vi "Set - wForm from Raw Data.vi"(0 "reference in":refnum<class "GSwFormDSP.lvclass">, 5 "error in (no error)":errorcluster, 6 "X Unit":string, 7 "Y Data (Row matrix)":dbl[][](array[numeric]), 8 "Data Origin":string, 9 "dTs":dbl[](array[numeric]), 10 "Signal Set":T1(ring), 11 "Signals Name":string[](array[string]), 13 "Signals Unit":string[](array[string])) -> (14 "reference in":refnum<class "GSwFormDSP.lvclass">, 19 "error out":errorcluster)   [LabVIEW 2020, in "GSwFormDSP.lvclass"]
uses:
  GSwFormDSP.lvclass
  functions/Attribute List.ctl
  Generic Utilities_class/Generic Utilities.lvclass
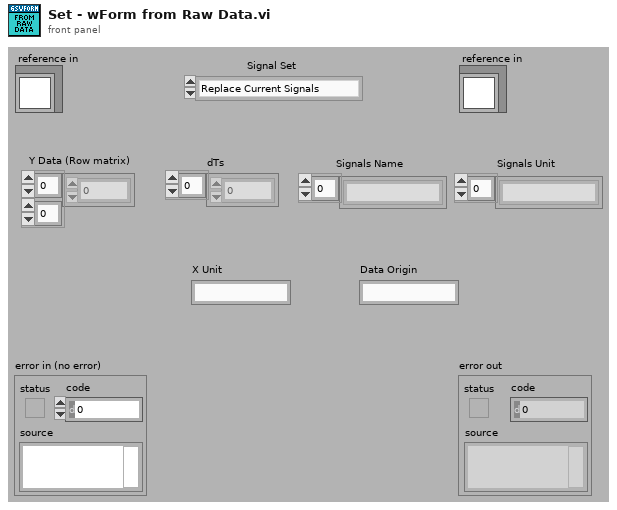
[diagram p1: front panel]
types:
  T1 = enum16{"Replace Current Signals", "Append to Current Signals"}
  T2 = typedef "GSwFormDSP.lvclass/Attribute List.ctl" = string
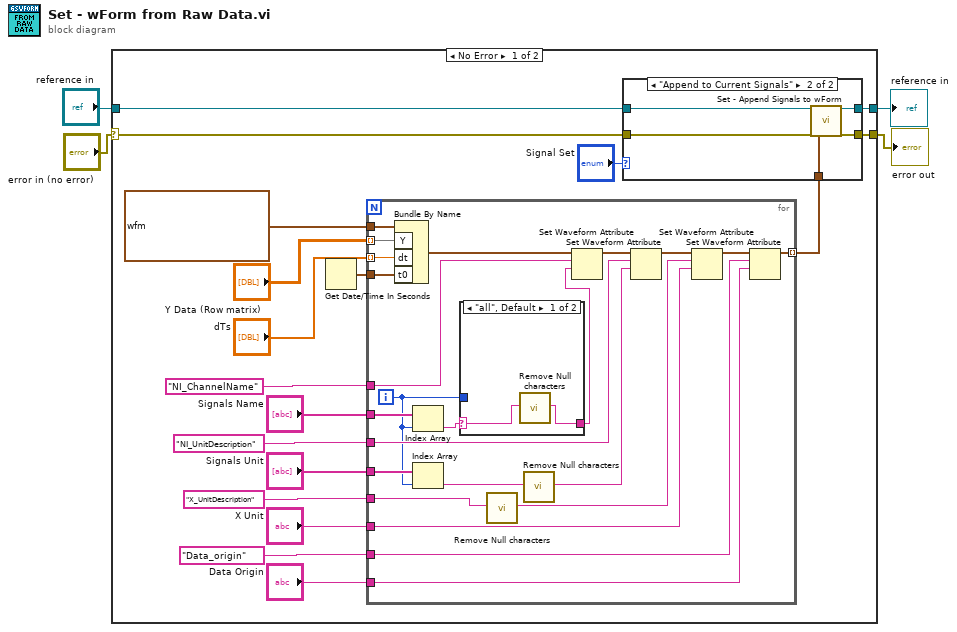
[diagram p0: block diagram]
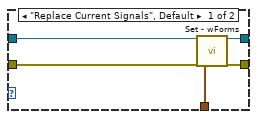
[diagram p2: hidden frame]
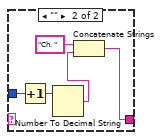
[diagram p3: hidden frame]
diagram:
  n1 = case shown="No Error" "error in (no error)" {
    selector: "error in (no error)" -> [w12 w64]
    tunnel: [w11 w64] -> w3
    tunnel: [w10 w63] -> w1
    tunnel: "reference in" -> [w14 w63]
    frame No Error {
      n2 = Get Date/Time In Seconds() -> (seconds since 1Jan1904=w17:timestamp)
      n3 = for {
        tunnel: waveform(dbl) {"t0"=timestamp(0 s since 1904-01-01), "dt"=1.0, "Y"=[]} ("Waveform") -> [w55]
        tunnel: "Y Data (Row matrix)" -> [w54] mode=indexing
        tunnel: "dTs" -> [w53] mode=indexing
        tunnel: w17 -> [w52]
        tunnel: T2 "NI_ChannelName" ("wForm Attributes") -> [w50]
        tunnel: "Signals Name" -> [w49]
        tunnel: "Signals Unit" -> [w48]
        tunnel: T2 "NI_UnitDescription" ("wForm Attributes") -> [w46]
        tunnel: T2 "X_UnitDescription" ("wForm Attributes") -> [w34]
        tunnel: "X Unit" -> [w44]
        tunnel: T2 "Data_origin" ("wForm Attributes") -> [w42]
        tunnel: "Data Origin" -> [w41]
        tunnel: [w40] -> w13 mode=indexing
        i -> [w37]
        n4 = Bundle By Name(cluster=w55, "Y"=w54, "dt"=w53, "t0"=w52) -> (w51:waveform(dbl))
        n5 = Index Array(array=w49, index=w37) -> (element=w39:string)
        n6 = Index Array(array=w48, index=w37) -> (element=w36:string)
        n7 = case shown="\"all\", Default" w39 {
          selector: w39 -> [w57 _]
          tunnel: [w56 w58] -> w38
          tunnel: w37 -> [_ w61]
          frame "all", Default {
            n8 = call "Remove Null characters.vi"("String IN"=w57) -> ("String OUT"=w56:string)  [unwired: 18 in]
          }
          frame "" {
            n9 = Increment(x=w61) -> (x+1=w62:i32)
            n10 = Number To Decimal String(number=w62) -> (decimal integer string=w59:string)  [unwired: 1 in]
            n11 = Concatenate Strings("Ch. " ("string"), w59) -> (w58:string)
          }
        }
        n12 = call "Remove Null characters.vi"("String IN"=w34) -> ("String OUT"=w33:string)  [unwired: 18 in]
        n13 = call "Remove Null characters.vi"("String IN"=w36) -> ("String OUT"=w35:string)  [unwired: 18 in]
        n14 = Set Waveform Attribute(5:w38, 6:w50, 7:w51) -> (3:w47:waveform(dbl))  [unwired: 1 in, 2 out]
        n15 = Set Waveform Attribute(5:w35, 6:w46, 7:w47) -> (3:w45:waveform(dbl))  [unwired: 1 in, 2 out]
        n16 = Set Waveform Attribute(5:w44, 6:w33, 7:w45) -> (3:w43:waveform(dbl))  [unwired: 1 in, 2 out]
        n17 = Set Waveform Attribute(5:w41, 6:w42, 7:w43) -> (3:w40:waveform(dbl))  [unwired: 1 in, 2 out]
      }
      n18 = case shown="\"Append to Current Signals\"" "Signal Set" {
        tunnel: w14 -> [w27 w32]
        tunnel: w13 -> [w26 w28]
        tunnel: w12 -> [w25 w31]
        tunnel: [w24 w29] -> w11
        tunnel: [w23 w30] -> w10
        frame "Replace Current Signals", Default {
          n19 = call "Set - wForms.vi"("reference in"=w27, "error in (no error)"=w25, "wForms"=w26) -> ("reference out"=w23:refnum<class "GSwFormDSP.lvclass">, "error out"=w24:errorcluster)  [unwired: 15 in]
        }
        frame "Append to Current Signals" {
          n20 = call "Set - Append Signals to wForm.vi"("reference in"=w32, "error in (no error)"=w31, "New Signals"=w28) -> ("reference out"=w30:refnum<class "GSwFormDSP.lvclass">, "error out"=w29:errorcluster)  [unwired: 15 in]
        }
      }
    }
    frame Error {
    }
  }
  "error out" <- w3
  "reference in" <- w1
